vi "Save Meta Data.vi"(6 "Channel name":string, 7 "Group name":string, 8 "Error In":errorcluster, 9 "Name":string, 10 "Value":variant, 11 "tdms file":refnum<k34>) -> (0 "Error Out":errorcluster, 3 "tdms file out":refnum<k34>)   [LabVIEW 2016]
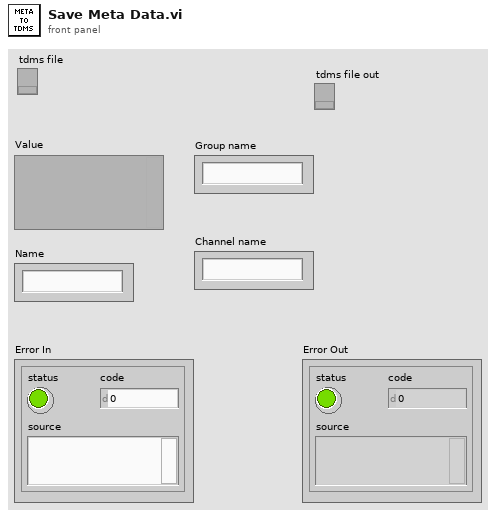
[diagram p1: front panel]
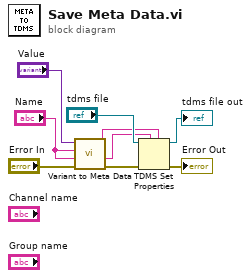
[diagram p0: block diagram]
diagram:
  n1 = call "Variant to Meta Data.vi"("Error In"="Error In", "Name"="Name", "key (optional)"="Name", "Value"="Value") -> ("Error Out"=w3:errorcluster, "Name out"=w4:string, "Meta data"=w5:string)  [unwired: 4 in, 1 out]
  n2 = TDMS Set Properties(5:w5, 7:w4, 8:w3, 11:"tdms file") -> (0:→"Error Out":errorcluster, 3:→"tdms file out":refnum<k34>)  [unwired: 2 in, 2 out]
